vi "Aurora Reader (Single Port) .vi"(2 "AXI4-Stream Reader FXP64x4":T1, 12 "ready for output":bool=TRUE) -> (4 "data":bool[](array[boolean]), 10 "output valid":bool)   [LabVIEW 2019]
uses:
  AXI4-Stream Reader FXP64x4 Resources.ctl
  <vilib>/rvi/eio/common/nirviEmuTemplateMethod_errors.vi
  <instrlib>/_niInstr/Data Formatting/v1/FPGA/Private/Convert/U64 array to Boolean Array.vi
  <instrlib>/_niInstr/Data Formatting/v1/FPGA/Private/Convert/U32 array to Boolean Array.vi
  <vilib>/eio/EIONode/EIONode.xnode
  <instrlib>/_niInstr/Basic Elements/v1/FPGA/niInstr Basic Elements v1 FPGA.lvlib
  <instrlib>/_niInstr/Data Formatting/v1/FPGA/niInstr Data Formatting v1 FPGA.lvlib
panel:
  out "tuser":bool[](array[boolean])
  out "tstrb":bool[](array[boolean])
  out "tkeep":bool[](array[boolean])
  out "tlast":bool
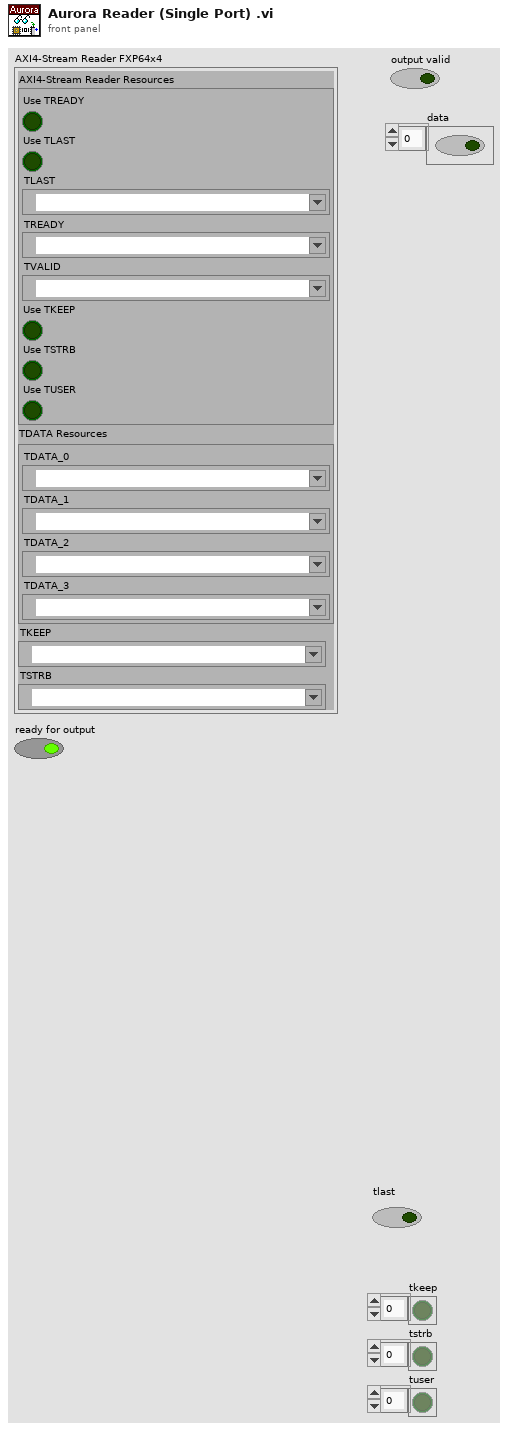
[diagram p1: front panel]
types:
  T1 = typedef "AXI4-Stream Reader FXP64x4 Resources.ctl" = cluster{"AXI4-Stream Reader Resources":cluster{"Use TREADY":bool, "Use TLAST":bool, "TLAST":refnum<k21>, "TREADY":refnum<k21>, "TVALID":refnum<k21>, "Use TKEEP":bool, "Use TSTRB":bool, "Use TUSER":bool}, "TDATA Resources":cluster{"TDATA_0":refnum<k21>, "TDATA_1":refnum<k21>, "TDATA_2":refnum<k21>, "TDATA_3":refnum<k21>}, "TKEEP":refnum<k21>, "TSTRB":refnum<k21>}
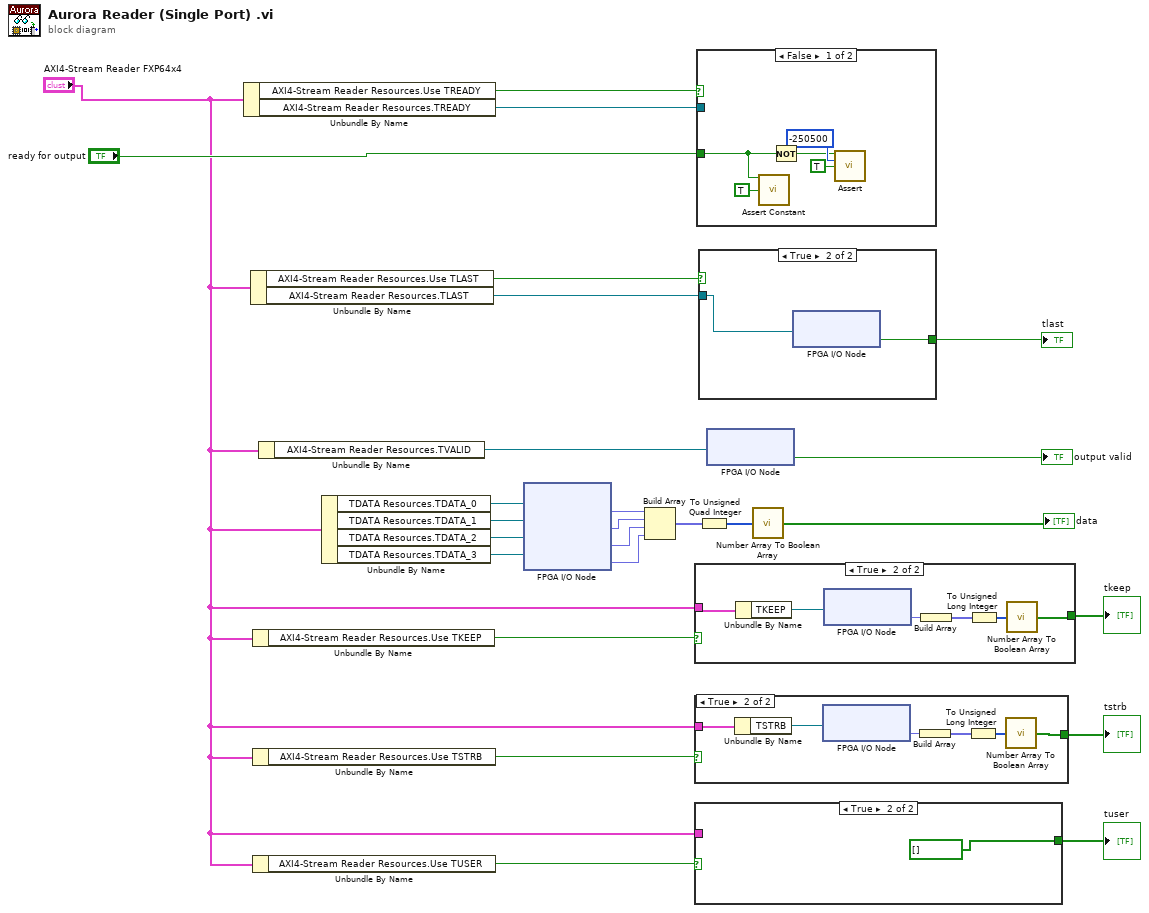
[diagram p0: block diagram]
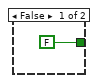
[diagram p5: hidden frame]
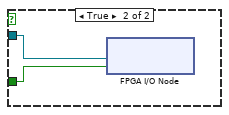
[diagram p6: hidden frame]
diagram:
  n1 = Unbundle By Name("AXI4-Stream Reader FXP64x4") -> ("AXI4-Stream Reader Resources.Use TREADY"=w26:bool, "AXI4-Stream Reader Resources.TREADY"=w25:refnum<k21>)
  n2 = Unbundle By Name("AXI4-Stream Reader FXP64x4") -> ("AXI4-Stream Reader Resources.Use TLAST"=w24:bool, "AXI4-Stream Reader Resources.TLAST"=w23:refnum<k21>)
  n3 = Unbundle By Name("AXI4-Stream Reader FXP64x4") -> ("AXI4-Stream Reader Resources.Use TKEEP"=w20:bool)
  n4 = Unbundle By Name("AXI4-Stream Reader FXP64x4") -> ("AXI4-Stream Reader Resources.Use TSTRB"=w18:bool)
  n5 = Unbundle By Name("AXI4-Stream Reader FXP64x4") -> ("AXI4-Stream Reader Resources.Use TUSER"=w16:bool)
  n6 = Unbundle By Name("AXI4-Stream Reader FXP64x4") -> ("AXI4-Stream Reader Resources.TVALID"=w21:refnum<k21>)
  n7 = Unbundle By Name("AXI4-Stream Reader FXP64x4") -> ("TDATA Resources.TDATA_0"=w12:refnum<k21>, "TDATA Resources.TDATA_1"=w11:refnum<k21>, "TDATA Resources.TDATA_2"=w10:refnum<k21>, "TDATA Resources.TDATA_3"=w9:refnum<k21>)
  n8 = xnode "FPGA I/O Node"("FPGA I/O In"=w12, "FPGA I/O In"=w11, "FPGA I/O In"=w10, "FPGA I/O In"=w9) -> ("I/O Item"=w8:fxp<+,64,64>, "I/O Item"=w7:fxp<+,64,64>, "I/O Item"=w6:fxp<+,64,64>, "I/O Item"=w5:fxp<+,64,64>)  [unwired: 4 out]
  n9 = Build Array(w8, w7, w6, w5) -> (w4:fxp<+,64,64>[])
  n10 = case shown="True" w20 {
    tunnel: "AXI4-Stream Reader FXP64x4" -> [_ w28]
    tunnel: [_ w27] -> w19
    frame False {
    }
    frame True {
      n11 = Unbundle By Name(w28) -> ("TKEEP"=w30:refnum<k21>)
      n12 = xnode "FPGA I/O Node"("FPGA I/O In"=w30) -> ("I/O Item"=w29:fxp<+,32,32>)  [unwired: 1 out]
      n13 = Build Array(w29) -> (w31:fxp<+,32,32>[])
      n14 = To Unsigned Long Integer(number=w31) -> (unsigned 32bit integer=w32:u32[])
      n15 = call-poly <instrlib>:"Number Array To Boolean Array.vi"("data in"=w32) -> ("data out"=w27:bool[])  [unwired: 14 in]
    }
  }
  "tkeep" <- w19
  n16 = case shown="True" w18 {
    tunnel: "AXI4-Stream Reader FXP64x4" -> [_ w34]
    tunnel: [_ w33] -> w17
    frame False {
    }
    frame True {
      n17 = Unbundle By Name(w34) -> ("TSTRB"=w37:refnum<k21>)
      n18 = xnode "FPGA I/O Node"("FPGA I/O In"=w37) -> ("I/O Item"=w38:fxp<+,32,32>)  [unwired: 1 out]
      n19 = Build Array(w38) -> (w36:fxp<+,32,32>[])
      n20 = To Unsigned Long Integer(number=w36) -> (unsigned 32bit integer=w35:u32[])
      n21 = call-poly <instrlib>:"Number Array To Boolean Array.vi"("data in"=w35) -> ("data out"=w33:bool[])  [unwired: 14 in]
    }
  }
  "tstrb" <- w17
  n22 = case shown="True" w16 {
    tunnel: "AXI4-Stream Reader FXP64x4" -> [_ _]
    tunnel: [_ bool[] [] ("value")] -> w15
    frame False {
    }
    frame True {
    }
  }
  "tuser" <- w15
  n23 = case shown="False" w26 {
    tunnel: w25 -> [_ w46]
    tunnel: "ready for output" -> [w43 w45]
    frame False {
      n24 = call <instrlib>:"Assert Constant.vi"("constant terminal"=w43, "enable show error"=TRUE) -> ()  [unwired: 14 in]
      n25 = Not(x=w43) -> (.not. x?=w40:bool)
      n26 = call <instrlib>:"Assert.vi"("assert"=w40, "error code"=-250500, "enable show error"=TRUE) -> ()  [unwired: 13 in]
    }
    frame True {
      n27 = xnode "FPGA I/O Node"("I/O Item"=w45, "FPGA I/O In"=w46) -> ()  [unwired: 1 out]
    }
  }
  n28 = case shown="True" w24 {
    tunnel: w23 -> [_ w49]
    tunnel: [FALSE ("I/O Item") w48] -> w22
    frame False {
    }
    frame True {
      n29 = xnode "FPGA I/O Node"("FPGA I/O In"=w49) -> ("I/O Item"=w48:bool)  [unwired: 1 out]
    }
  }
  "tlast" <- w22
  n30 = To Unsigned Quad Integer(1:w4) -> (0:w3:u64[])
  n31 = xnode "FPGA I/O Node"("FPGA I/O In"=w21) -> ("I/O Item"=→"output valid":bool)  [unwired: 1 out]
  n32 = call-poly <instrlib>:"Number Array To Boolean Array.vi"("data in"=w3) -> ("data out"=→"data":bool[])  [unwired: 14 in]
